vi "point-by-point torque with filtering duplicate.vi"(6 "encoders offset":u32 caption="encoder offset @ 1Hz (ticks)", 8 "speed history in":u32[](array[numeric])=[0, 0, 0, 0, 0, 0, 0, 0, 0, 0, 0, 0, 0, 0, 0, 0, 0, 0, 0, 0, 0, 0, 0, 0, 0, 0, 0, 0, 0, 0, 0, 0, 0, 0, 0, 0, 0, 0, 0, 0], 9 "torque history":i32[](array[numeric])=[0, 0, 0, 0, 0, 0, 0, 0, 0, 0, 0, 0, 0, 0, 0, 0, 0, 0, 0, 0, 0, 0, 0, 0, 0, 0, 0, 0, 0, 0, 0, 0, 0, 0, 0, 0, 0, 0, 0, 0], 10 "angle pulse":u32, 11 "speed pulse":u32) -> (0 "speed history out":u32[](array[numeric]), 1 "torque history out":i32[](array[numeric]), 2 "calculated angle (degrees)":sgl, 3 "calculated speed (Hz)":sgl, 4 "measured encoder delta":sgl)   [LabVIEW 2018]
panel:
  out "mean delta":sgl
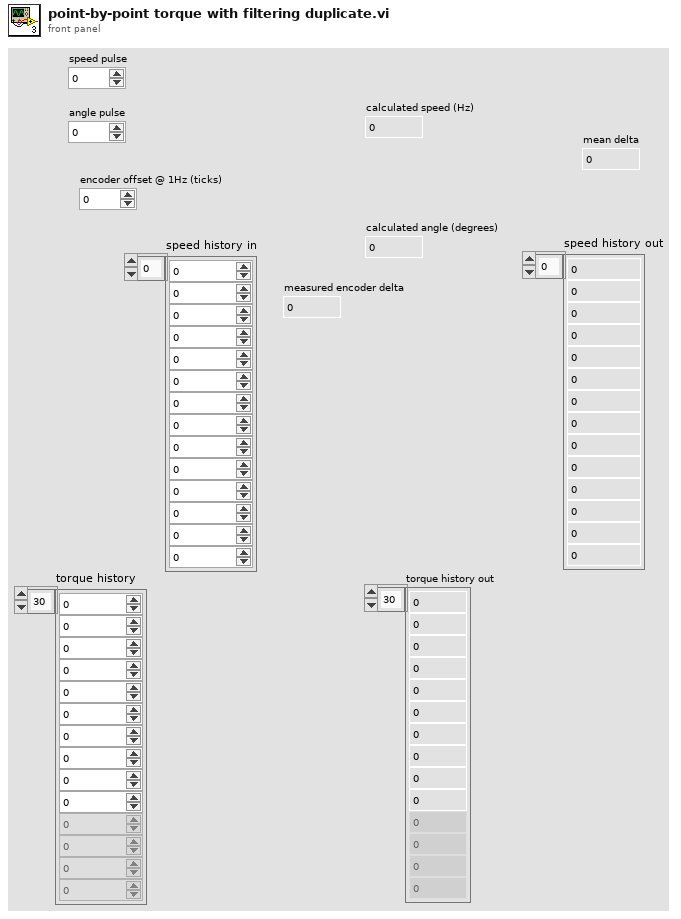
[diagram p1: front panel]
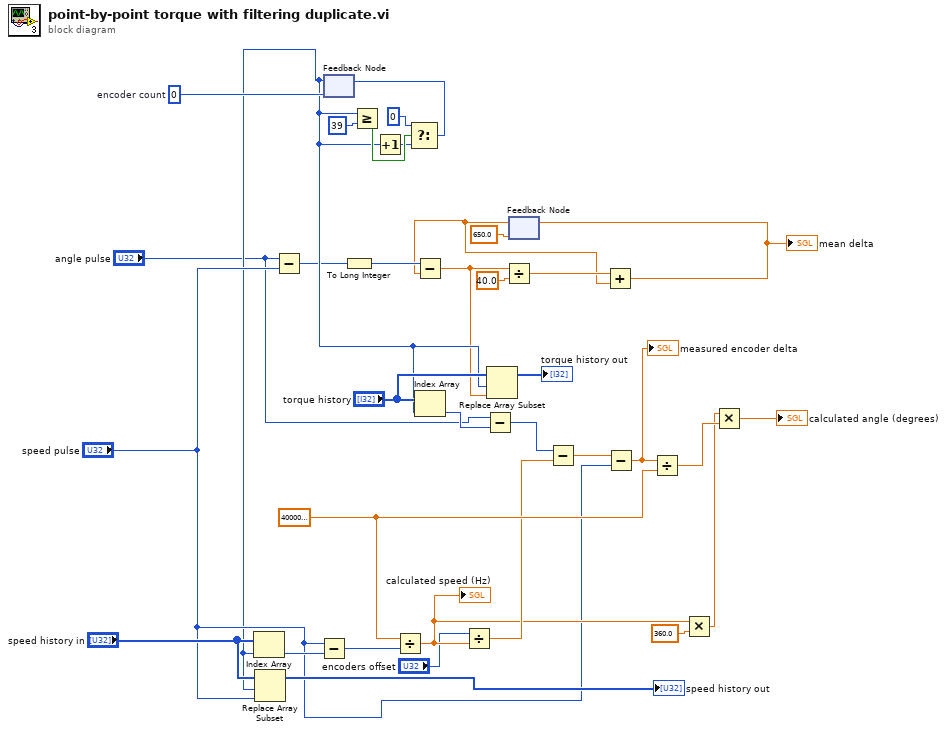
[diagram p0: block diagram]
diagram:
  w19 = 0  # encoder count
  w30 = sgl 40000000.0 ("64bit integer")
  n1 = Subtract(x="angle pulse", y="speed pulse") -> (x-y=w2:u32)
  n2 = feedback #1(w19) -> (w7:i32)
  n3 = Index Array(array="speed history in", index=w7) -> (element=w35:u32)
  n4 = Replace Array Subset(array="speed history in", new element="speed pulse", index=w7) -> (→"speed history out":u32[])
  n5 = Subtract(x="speed pulse", y=w35) -> (x-y=w34:u32)
  n6 = To Long Integer(number=w2) -> (32bit integer=w13:i32)
  n7 = Greater Or Equal?(x=w7, y=39) -> (x >= y?=w22:bool)
  n8 = Increment(x=w7) -> (x+1=w21:i32)
  n9 = Divide(x=w30, y=w34) -> (x/y=w25:sgl)
  "calculated speed (Hz)" <- w25
  n10 = Select(t=0, s=w22, f=w21) -> (s? t:f=w18:i32)
  n11 = feedback-in #1(w18) -> ()
  n12 = Index Array(array="torque history", index=w7) -> (element=w5:i32)
  n13 = Divide(x="encoders offset", y=w25) -> (x/y=w26:sgl)
  n14 = Subtract(x="angle pulse", y=w5) -> (x-y=w4:u32)
  n15 = feedback #2(sgl 650.0) -> (w10:sgl)
  n16 = Subtract(x=w13, y=w10) -> (x-y=w6:sgl)
  n17 = Replace Array Subset(array="torque history", new element=w6, index=w7) -> (→"torque history out":i32[])
  n18 = Divide(x=w6, y=sgl 40.0) -> (x/y=w12:sgl)
  n19 = Subtract(x=w4, y=w26) -> (x-y=w33:sgl)
  n20 = Add(x=w12, y=w10) -> (x+y=w11:sgl)
  "mean delta" <- w11
  n21 = feedback-in #2(w11) -> ()
  n22 = Subtract(x=w33, y="speed pulse") -> (x-y=w31:sgl)
  "measured encoder delta" <- w31
  n23 = Divide(x=w31, y=w30) -> (x/y=w29:sgl)
  n24 = Multiply(x=w25, y=sgl 360.0) -> (x*y=w28:sgl)
  n25 = Multiply(x=w28, y=w29) -> (x*y=→"calculated angle (degrees)":sgl)
